vi "Channel1_control.vi"(4 "Auto adjust ON":bool, 6 "V/DIV 1":dbl, 7 "Measured frequency":dbl, 9 "S/DIV 1":dbl, 10 "Measured amplitude":dbl, 11 "WaveformGraph in":refnum<vi>) -> (2 "V/DIV out":string, 3 "S/DIV out":string)   [LabVIEW 2019]
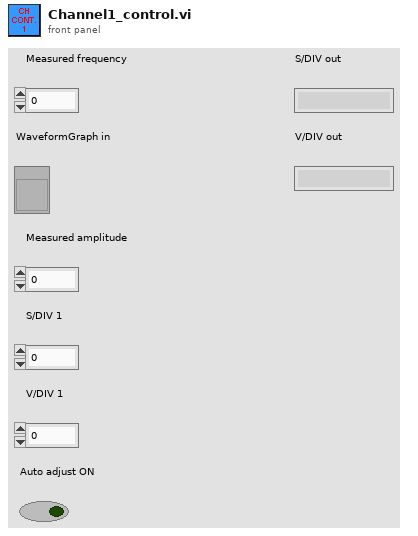
[diagram p1: front panel]
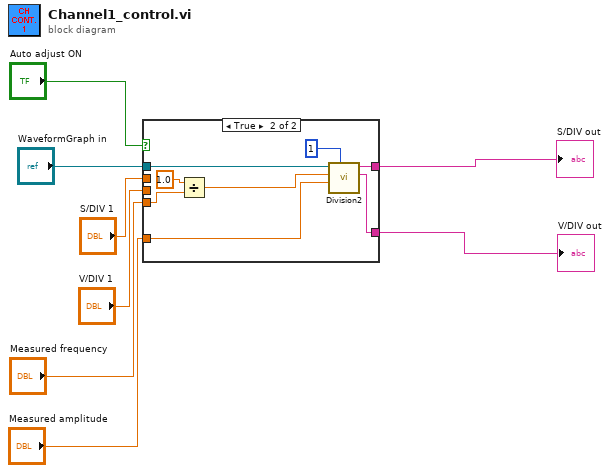
[diagram p0: block diagram]
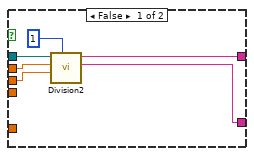
[diagram p2: hidden frame]
diagram:
  n1 = case shown="True" "Auto adjust ON" {
    tunnel: "WaveformGraph in" -> [w12 w22]
    tunnel: "S/DIV 1" -> [w11 _]
    tunnel: "V/DIV 1" -> [w10 _]
    tunnel: "Measured amplitude" -> [_ w19]
    tunnel: [w14 w18] -> w3
    tunnel: [w13 w17] -> w4
    tunnel: "Measured frequency" -> [_ w15]
    frame False {
      n2 = call "Division2.vi"("Scale_select"=u32 1, "V/div"=w10, "s/div"=w11, "WaveformGraph in"=w12) -> ("V/DIV"=w13:string, "S/DIV"=w14:string)  [unwired: 5 in, 1 out]
    }
    frame True {
      n3 = Divide(x=1.0, y=w15) -> (x/y=w21:dbl)
      n4 = call "Division2.vi"("Scale_select"=u32 1, "V/div"=w19, "s/div"=w21, "WaveformGraph in"=w22) -> ("V/DIV"=w17:string, "S/DIV"=w18:string)  [unwired: 5 in, 1 out]
    }
  }
  "V/DIV out" <- w4
  "S/DIV out" <- w3
